vi "MGCC_FntStaMach_StateCalculandEnableFlagCalcul.vi"(7 "ABN State Input":string[](array[string]), 8 "Error Input":errorcluster[](array[cluster]), 9 "ABN State input enable":bool[][](array[boolean]), 10 "Current State":string[](array[string]), 11 "Input Events":bool[][](array[boolean])) -> (0 "Error output":errorcluster[](array[cluster]), 1 "Next State":string[](array[string]), 2 "ABN State output":string[](array[string]), 3 "ABN Function Enable output":bool[][](array[boolean]), 4 "Function Enable 2":bool[][](array[boolean]), 5 "Function Enable 1":bool[][](array[boolean]))   [LabVIEW 2016]
uses:
  MGCC_FntStaMach_gobal.vi
  <vilib>/imath/engines/lvmath2/RunTimeEngine/IndexRead/NIMS V(S).vi
  <instcachedir>/0/NIMS V(S)_0488751826AF41519A22953C041130DC.lvgen/NIMS V(S)_0488751826AF41519A22953C041130DC_003.vi
  <vilib>/imathl/engines/lvmath/Functions/Error Handling/Create Error.vi
  <vilib>/imath/engines/lvmath2/RunTimeEngine/NodeEndStatement/NIMS_NodeEndStatement_Output.vi
  <instcachedir>/0/NIMS_NodeEndStatement_Output_53EC0D466D134D7ABD903AC30B43404B.lvgen/NIMS_NodeEndStatement_Output_53EC0D466D134D7ABD903AC30B43404B_011.vi
  <vilib>/imath/engines/lvmath2/RunTimeEngine/ErrorHandling/NIMS_Finalize Error.vi
panel:
  out "error out":errorcluster
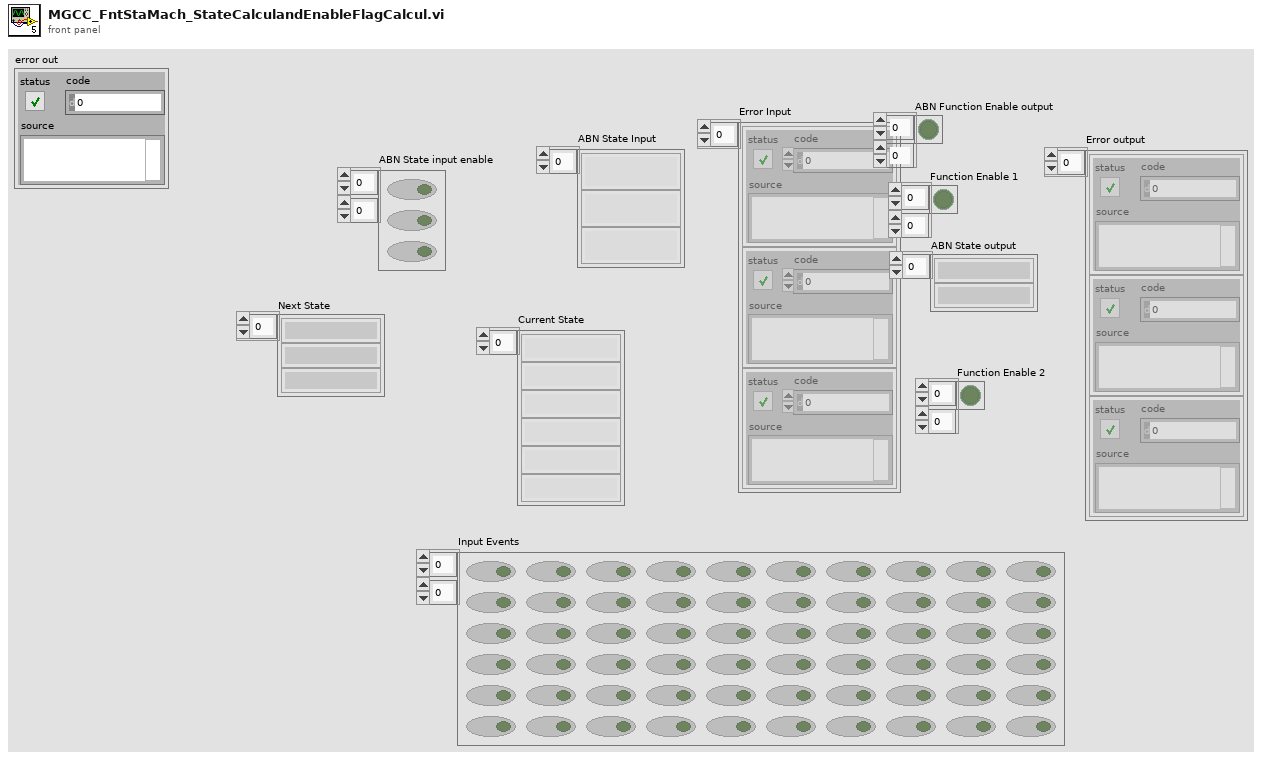
[diagram p1: front panel]
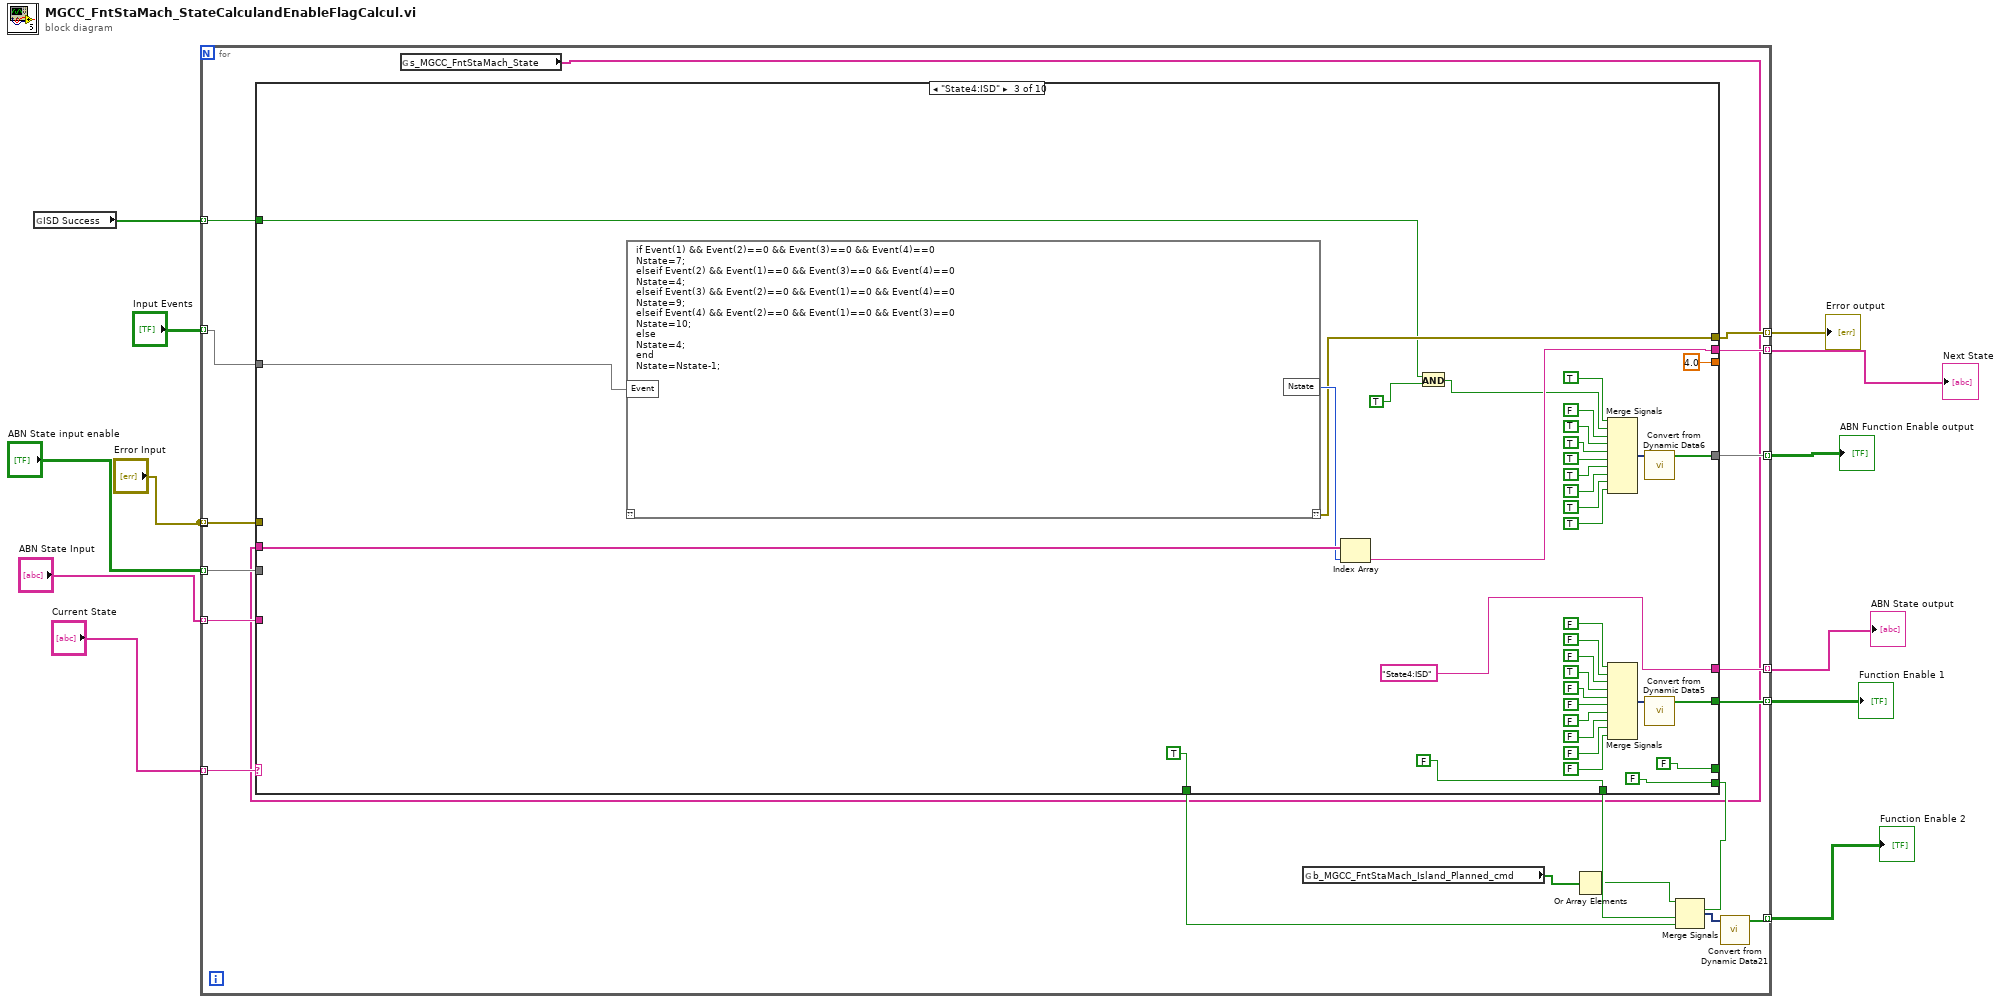
[diagram p0: block diagram]
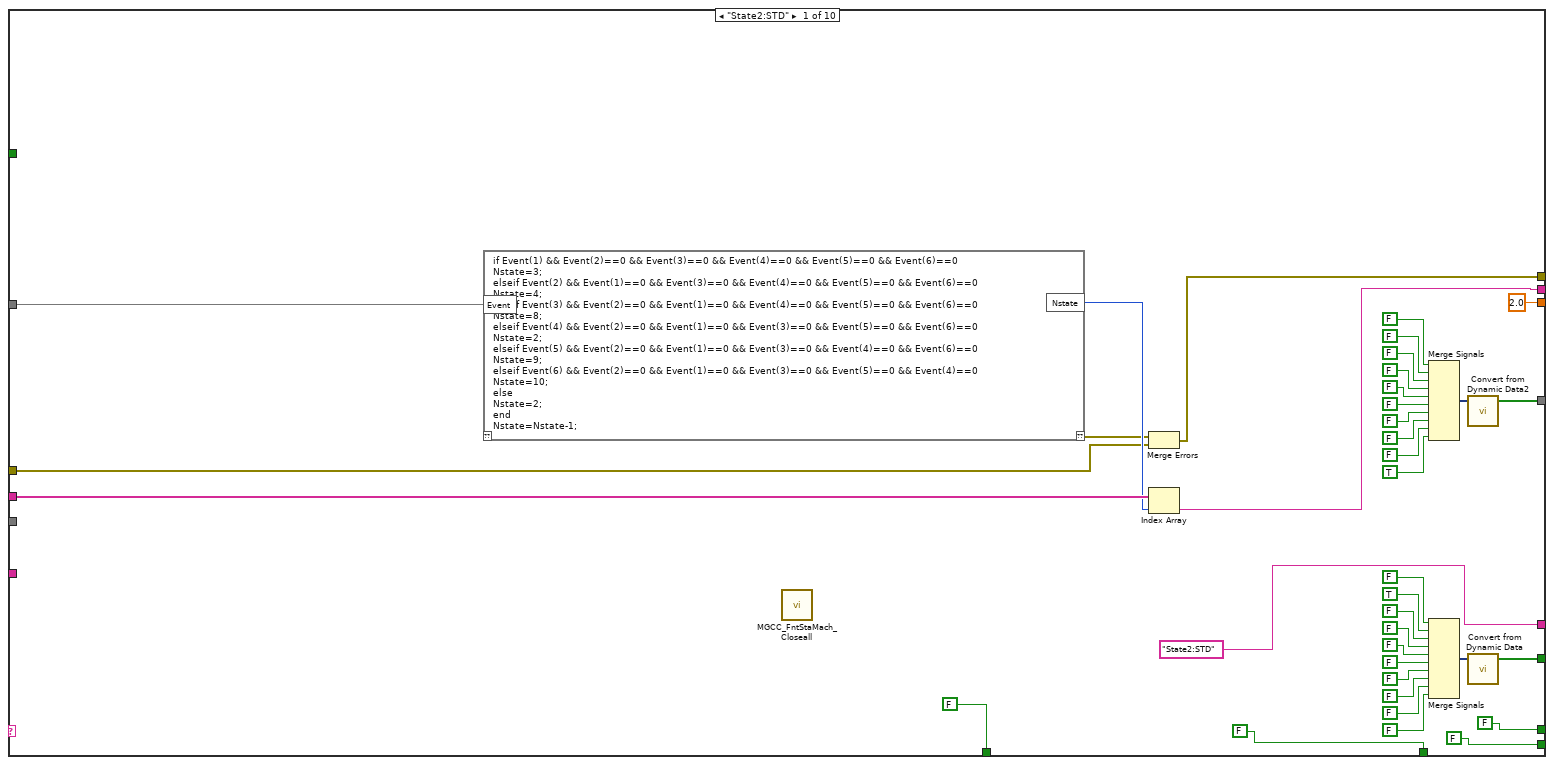
[diagram p2: hidden frame]
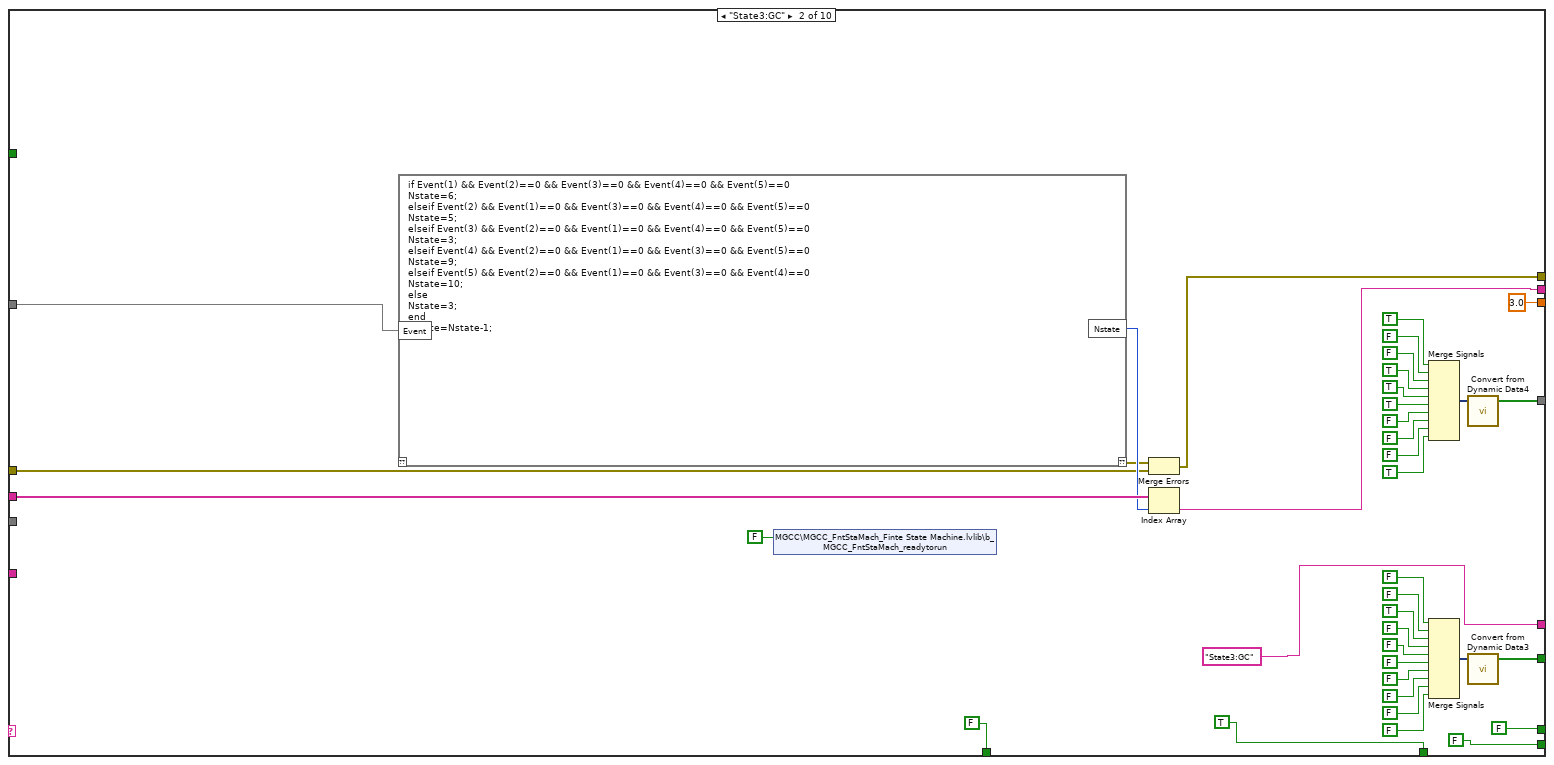
[diagram p3: hidden frame]
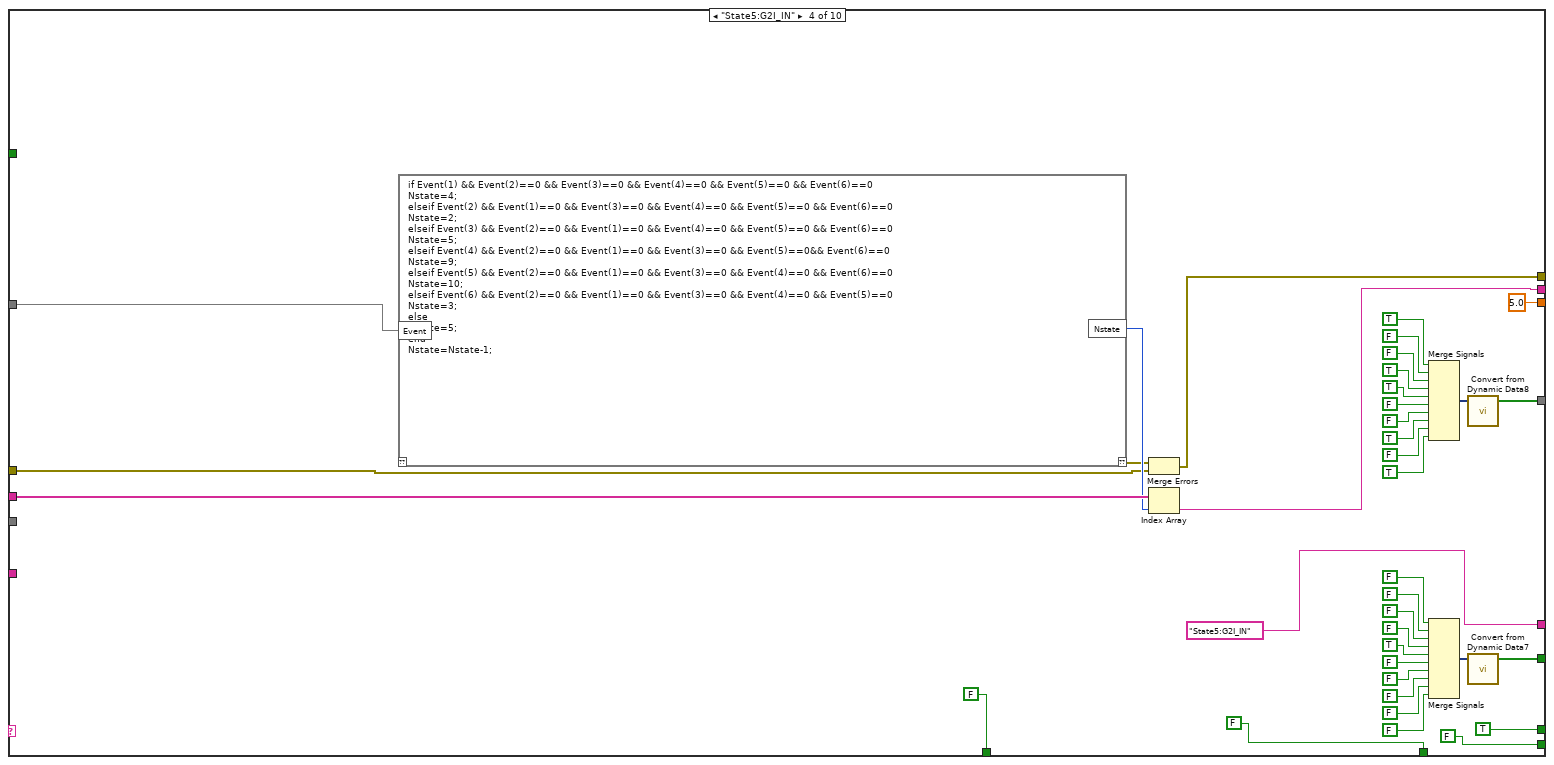
[diagram p4: hidden frame]
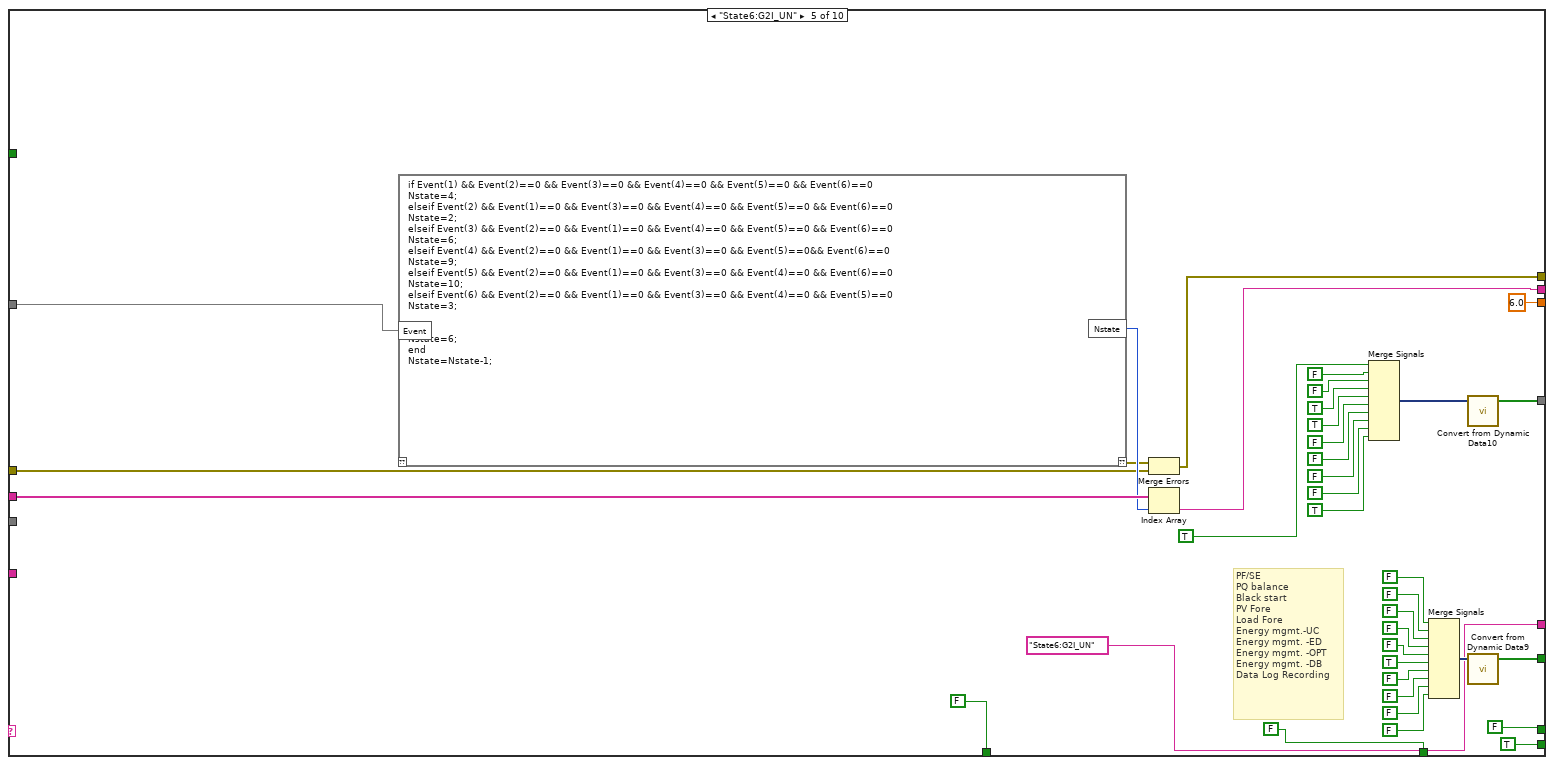
[diagram p5: hidden frame]
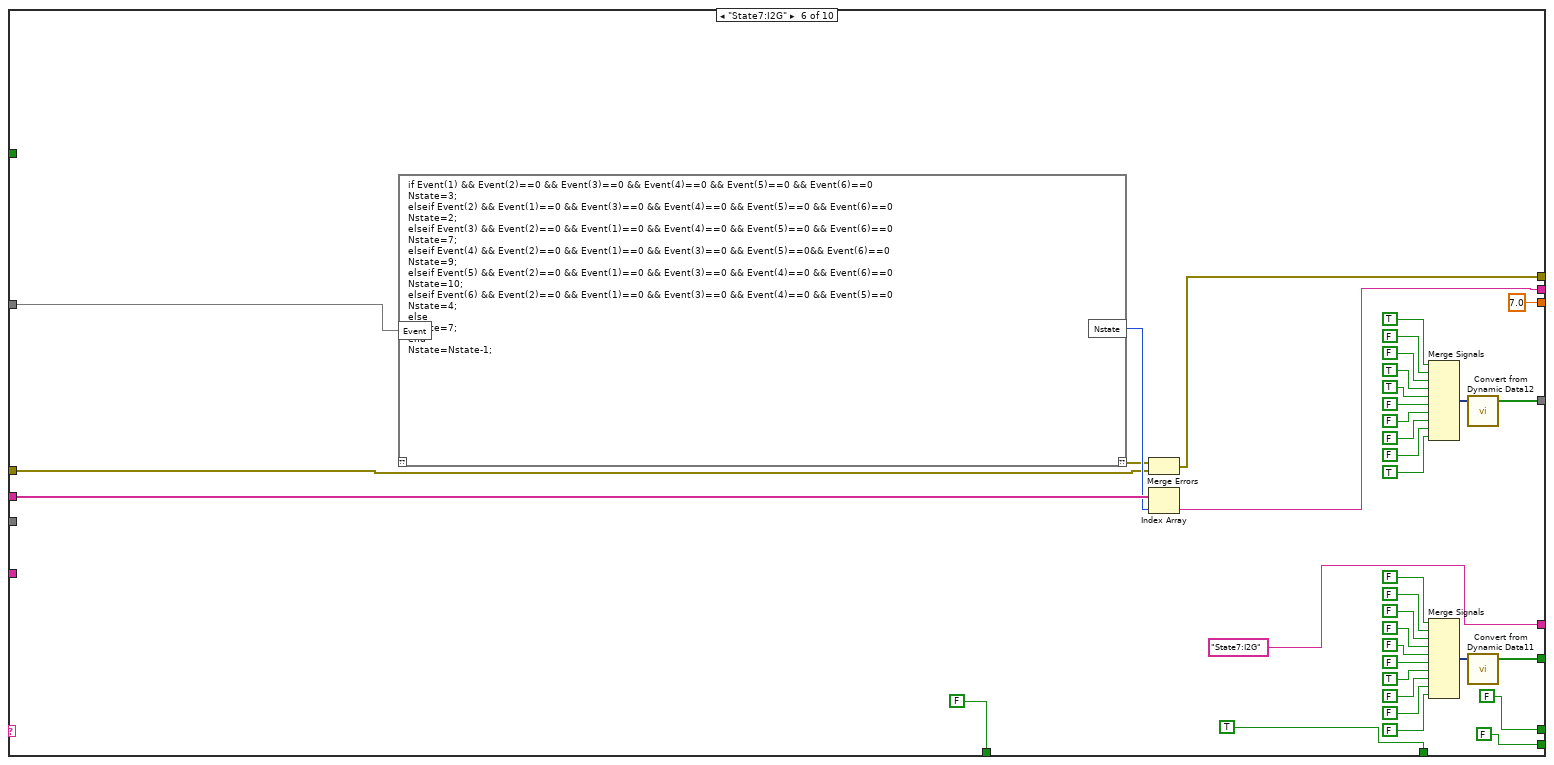
[diagram p6: hidden frame]
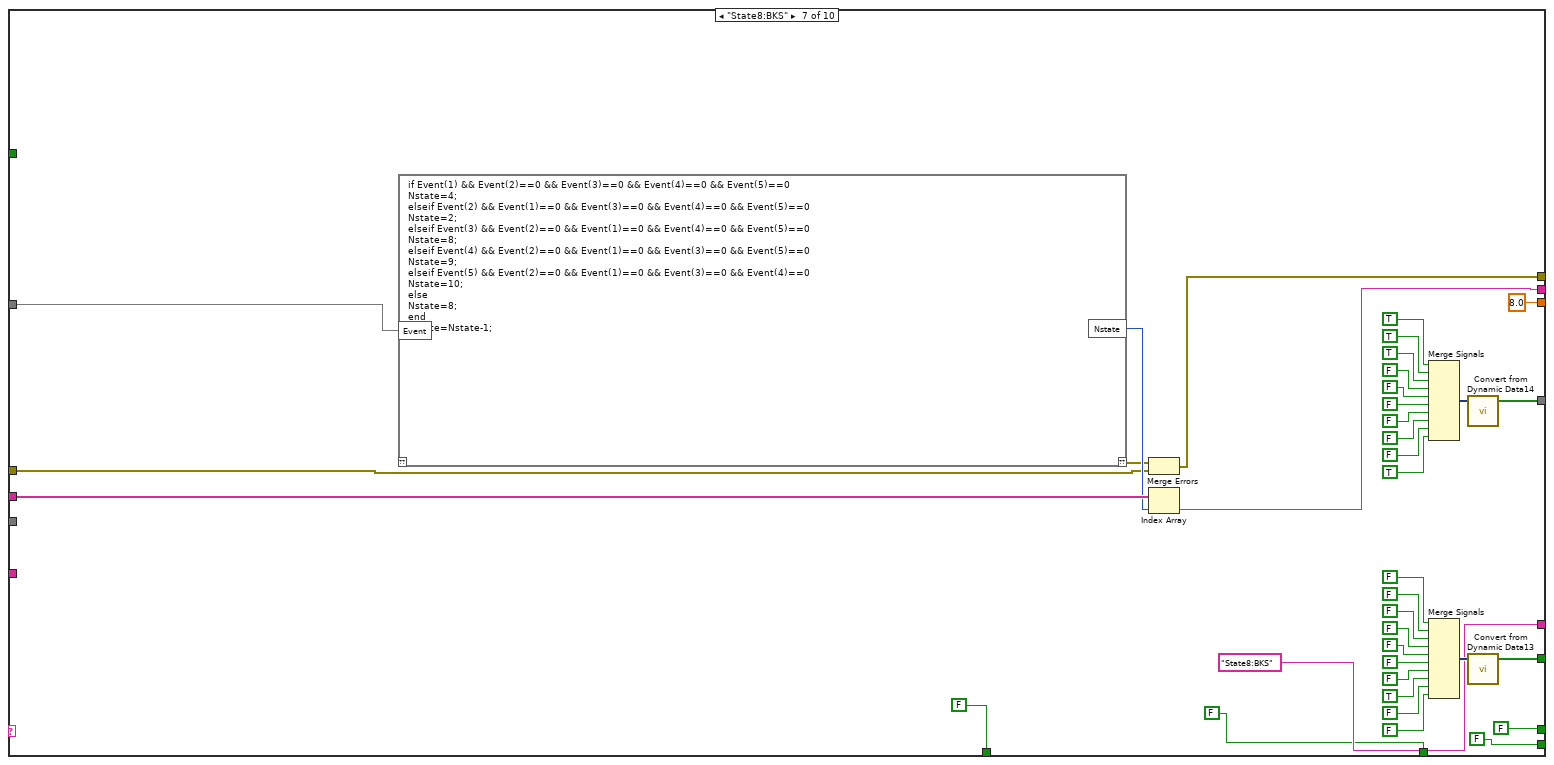
[diagram p7: hidden frame]
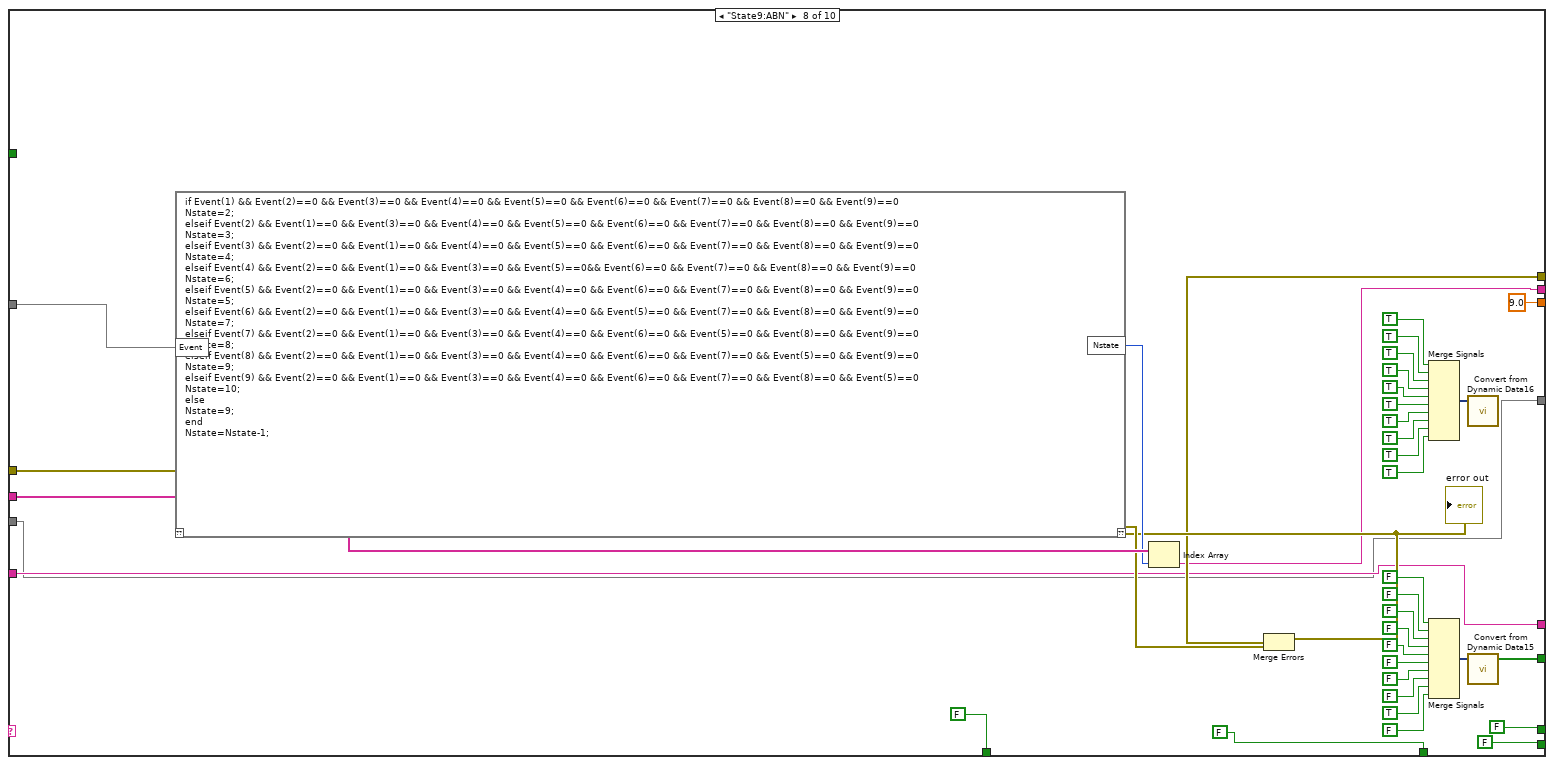
[diagram p8: hidden frame]
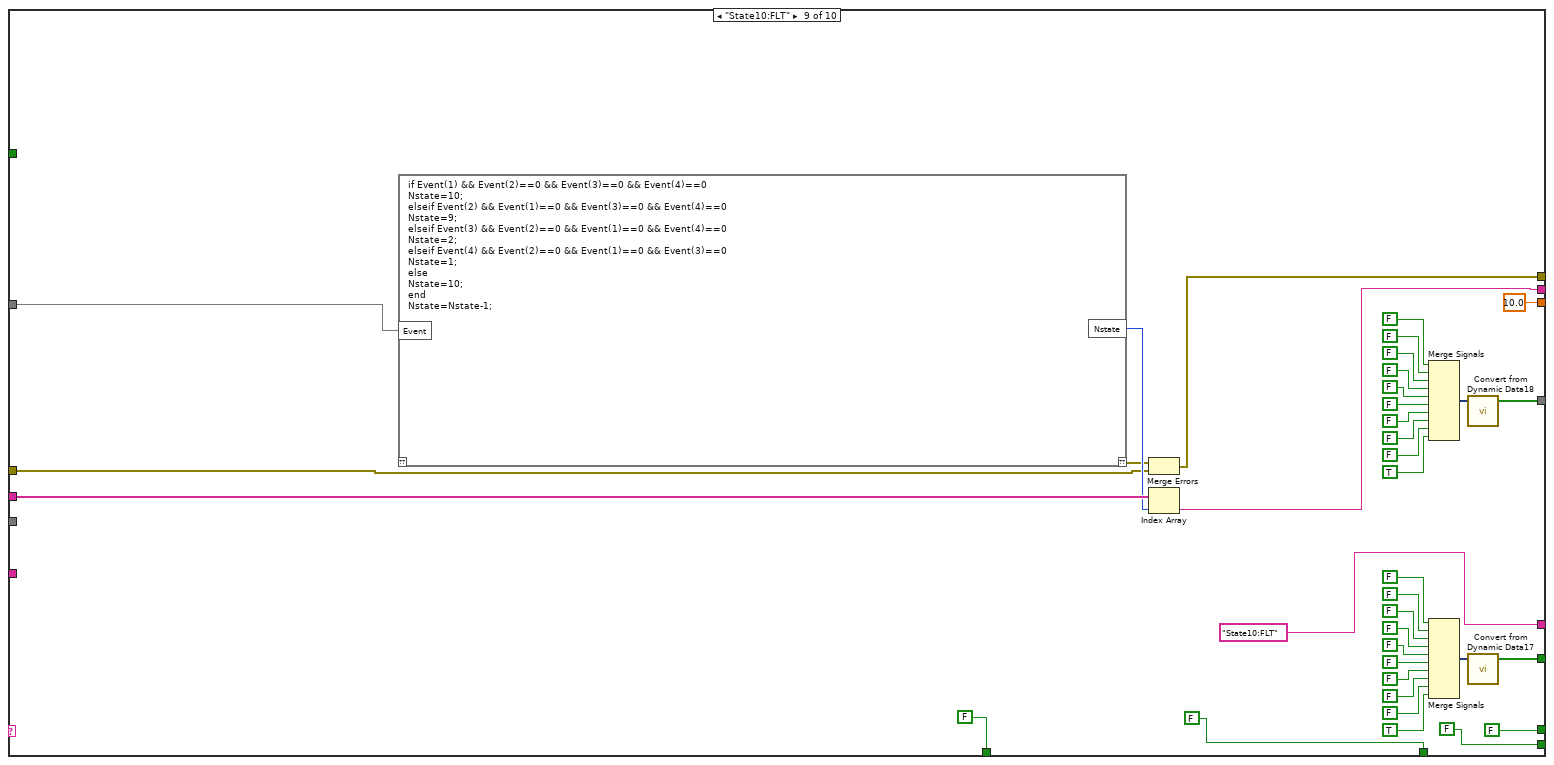
[diagram p9: hidden frame]
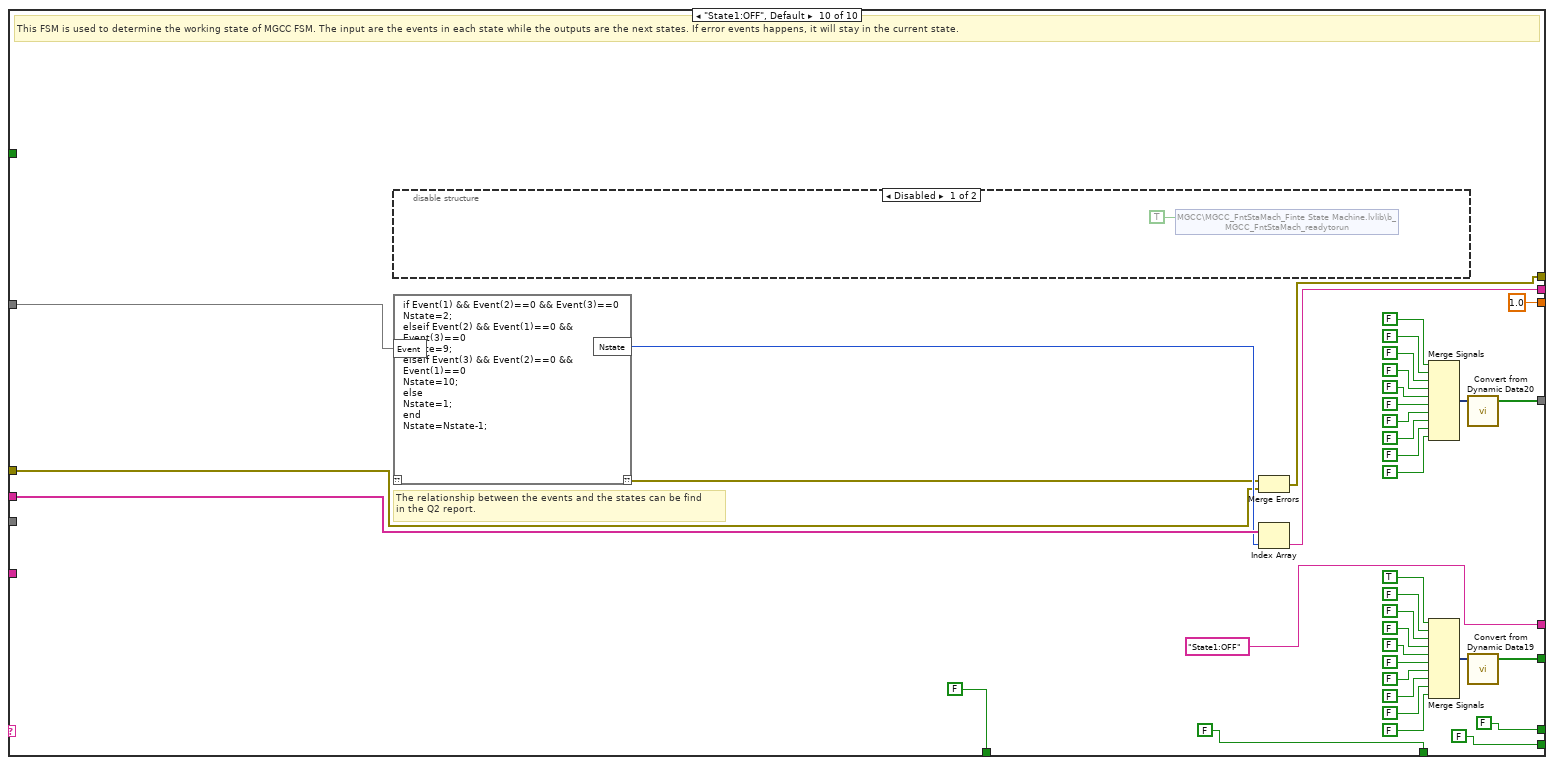
[diagram p10: hidden frame]
diagram:
  n1 = global read "MGCC_FntStaMach_gobal.vi" "ISD Success"() -> (w1:bool[])
  n2 = for {
    tunnel: "Input Events" -> [w30] mode=indexing
    tunnel: "Current State" -> [w31] mode=indexing
    tunnel: [w29] -> w10 mode=indexing
    tunnel: "Error Input" -> [_] mode=indexing
    tunnel: "Error Input" -> [w28] mode=indexing
    tunnel: [w27] -> w8 mode=indexing
    tunnel: [w26] -> w7 mode=indexing
    tunnel: "ABN State Input" -> [w25] mode=indexing
    tunnel: [w24] -> w5 mode=indexing
    tunnel: "ABN State input enable" -> [w23] mode=indexing
    tunnel: [w22] -> w3 mode=indexing
    tunnel: [w17] -> w2 mode=indexing
    tunnel: w1 -> [w15] mode=indexing
    n3 = global read "MGCC_FntStaMach_gobal.vi" "s_MGCC_FntStaMach_State"() -> (w16:string[])
    n4 = case shown="\"State4:ISD\"" w31 {
      tunnel: [w36 w1024 w1737 w2211 w3199 w4187 w5175 w5885 w8012 w8489] -> w22
      tunnel: [w57 w1046 w1754 w2232 w3220 w4208 w5196 w5904 w8032 w8510] -> w26
      tunnel: w16 -> [w56 w1045 w1753 w2231 w3219 w4207 w5195 w5903 w8031 w8509]
      tunnel: [w44 w1033 w1742 w2219 w3207 w4195 w5184 w5879 w8019 w8497] -> w27
      tunnel: [2.0 ("MS_Analog_Control_OS2_6") 3.0 ("MS_Analog_Control_OS2_6") 4.0 ("MS_Analog_Control_OS2_6") 5.0 ("MS_Analog_Control_OS2_6") 6.0 ("MS_Analog_Control_OS2_6") 7.0 ("MS_Analog_Control_OS2_6") 8.0 ("MS_Analog_Control_OS2_6") 9.0 ("MS_Analog_Control_OS2_6") 10.0 ("MS_Analog_Control_OS2_6") 1.0 ("MS_Analog_Control_OS2_6")] -> _
      tunnel: w30 -> [w41 w1029 w1739 w2216 w3204 w4192 w5180 w5889 w8016 w8494]
      tunnel: w28 -> [w40 w1028 _ w2215 w3203 w4191 w5179 w5888 w8015 w8493]
      tunnel: [w38 w1026 w1732 w2213 w3201 w4189 w5177 w5886 w8013 w8491] -> w29
      tunnel: ["State2:STD" "State3:GC" "State4:ISD" "State5:G2I_IN" "State6:G2I_UN" "State7:I2G" "State8:BKS" w5880 "State10:FLT" "State1:OFF"] -> w24
      tunnel: [FALSE ("State3") FALSE ("State3") FALSE ("State3") TRUE ("State3") FALSE ("State3") FALSE ("State3") FALSE ("State3") FALSE ("State3") FALSE ("State3") FALSE ("State3")] -> _
      tunnel: [FALSE ("State3") FALSE ("State3") FALSE ("State3") FALSE ("State3") TRUE ("State3") FALSE ("State3") FALSE ("State3") FALSE ("State3") FALSE ("State3") FALSE ("State3")] -> w21
      tunnel: [FALSE ("State3") TRUE ("State3") FALSE ("State3") FALSE ("State3") FALSE ("State3") TRUE ("State3") FALSE ("State3") FALSE ("State3") FALSE ("State3") FALSE ("State3")] -> w20
      tunnel: [FALSE ("State3") FALSE ("State3") TRUE ("State3") FALSE ("State3") FALSE ("State3") FALSE ("State3") FALSE ("State3") FALSE ("State3") FALSE ("State3") FALSE ("State3")] -> w19
      tunnel: w25 -> [_ _ _ _ _ _ _ w5880 _ _]
      tunnel: w23 -> [_ _ _ _ _ _ _ w5879 _ _]
      tunnel: w15 -> [_ _ w1731 _ _ _ _ _ _ _]
      frame "State2:STD" {
        n5 = mathscript code="if Event(1) && Event(2)==0 && Event(3)==0 && Event(4)==0 && Event(5)==0 && Event(6)==0\nNstate=3;\nelseif Event(2) && Event(1)==0 && Event(3)==0 && Event(4)==0 && Event(5)==0 && Event(6)==0\nNstate=4;\nelseif Event(3) && Event(2)==0 && Event(1)==0 && Event(4)==0 && Event(5)==0 && Event(6)==0\nNstate=8;\nelseif Event(4) && Event(2)==0 && Event(1)==0 && Event(3)==0 && Event(5)==0 && Event(6)==0\nNstate=2;\nelseif Event(5) && Event(2)==0 && Event(1)==0 && Event(3)==0 && Event(4)==0 && Event(6)==0\nNstate=9;\nelseif Event(6) && Event(2)==0 && Event(1)==0 && Event(3)==0 && Event(5)==0 && Event(4)==0\nNstate=10;\nelse\nNstate=2;\nend\nNstate=Nstate-1;"("Event"=w41) -> ("??"=w39:errorcluster, "Nstate"=w55:i32)  [unwired: 1 in]
        n6 = call "MGCC_FntStaMach_Closeall.vi"() -> ()  [unwired: 12 in]
        n7 = Merge Errors(w39, w40) -> (w38:errorcluster)
        n8 = Index Array(array=w56, index=w55) -> (element=w36:string)
        n9 = Merge Signals(FALSE ("State3"), FALSE ("State3"), FALSE ("State3"), FALSE ("State3"), FALSE ("State3"), FALSE ("State3"), FALSE ("State3"), FALSE ("State3"), FALSE ("State3"), TRUE ("State3")) -> (w45:dynamicdata)
        n10 = Merge Signals(FALSE ("State3"), TRUE ("State3"), FALSE ("State3"), FALSE ("State3"), FALSE ("State3"), FALSE ("State3"), FALSE ("State3"), FALSE ("State3"), FALSE ("State3"), FALSE ("State3")) -> (w58:dynamicdata)
        n11 = call "Convert from Dynamic Data2"("Dynamic Data Type"=w45) -> ("Array"=w44:bool[])  [unwired: 3 in]
        n12 = call "Convert from Dynamic Data"("Dynamic Data Type"=w58) -> ("Array"=w57:bool[])  [unwired: 3 in]
      }
      frame "State3:GC" {
        n13 = mathscript code="if Event(1) && Event(2)==0 && Event(3)==0 && Event(4)==0 && Event(5)==0 \nNstate=6;\nelseif Event(2) && Event(1)==0 && Event(3)==0 && Event(4)==0 && Event(5)==0 \nNstate=5;\nelseif Event(3) && Event(2)==0 && Event(1)==0 && Event(4)==0 && Event(5)==0 \nNstate=3;\nelseif Event(4) && Event(2)==0 && Event(1)==0 && Event(3)==0 && Event(5)==0\nNstate=9;\nelseif Event(5) && Event(2)==0 && Event(1)==0 && Event(3)==0 && Event(4)==0 \nNstate=10;\nelse\nNstate=3;\nend\nNstate=Nstate-1;"("Event"=w1029) -> ("??"=w1027:errorcluster, "Nstate"=w1044:i32)  [unwired: 1 in]
        n14 = shared-variable "MGCC\\MGCC_FntStaMach_Finte State Machine.lvlib\\b_MGCC_FntStaMach_readytorun"(FALSE ("b_MGCC_DataLog_enable")) -> ()  [unwired: 1 in, 1 out]
        n15 = Merge Errors(w1027, w1028) -> (w1026:errorcluster)
        n16 = Index Array(array=w1045, index=w1044) -> (element=w1024:string)
        n17 = Merge Signals(TRUE ("State3"), FALSE ("State3"), FALSE ("State3"), TRUE ("State3"), TRUE ("State3"), TRUE ("State3"), FALSE ("State3"), FALSE ("State3"), FALSE ("State3"), TRUE ("State3")) -> (w1034:dynamicdata)
        n18 = Merge Signals(FALSE ("State3"), FALSE ("State3"), TRUE ("State3"), FALSE ("State3"), FALSE ("State3"), FALSE ("State3"), FALSE ("State3"), FALSE ("State3"), FALSE ("State3"), FALSE ("State3")) -> (w1047:dynamicdata)
        n19 = call "Convert from Dynamic Data4"("Dynamic Data Type"=w1034) -> ("Array"=w1033:bool[])  [unwired: 3 in]
        n20 = call "Convert from Dynamic Data3"("Dynamic Data Type"=w1047) -> ("Array"=w1046:bool[])  [unwired: 3 in]
      }
      frame "State4:ISD" {
        n21 = mathscript code="if Event(1) && Event(2)==0 && Event(3)==0 && Event(4)==0 \nNstate=7;\nelseif Event(2) && Event(1)==0 && Event(3)==0 && Event(4)==0 \nNstate=4;\nelseif Event(3) && Event(2)==0 && Event(1)==0 && Event(4)==0 \nNstate=9;\nelseif Event(4) && Event(2)==0 && Event(1)==0 && Event(3)==0 \nNstate=10;\nelse\nNstate=4;\nend\nNstate=Nstate-1;"("Event"=w1739) -> ("??"=w1732:errorcluster, "Nstate"=w1752:i32)  [unwired: 1 in]
        n22 = Index Array(array=w1753, index=w1752) -> (element=w1737:string)
        n23 = And(x=w1731, y=TRUE ("State3")) -> (x .and. y?=w1729:bool)
        n24 = Merge Signals(TRUE ("State3"), w1729, FALSE ("State3"), TRUE ("State3"), TRUE ("State3"), TRUE ("State3"), TRUE ("State3"), TRUE ("State3"), TRUE ("State3"), TRUE ("State3")) -> (w1743:dynamicdata)
        n25 = Merge Signals(FALSE ("State3"), FALSE ("State3"), FALSE ("State3"), TRUE ("State3"), FALSE ("State3"), FALSE ("State3"), FALSE ("State3"), FALSE ("State3"), FALSE ("State3"), FALSE ("State3")) -> (w1755:dynamicdata)
        n26 = call "Convert from Dynamic Data6"("Dynamic Data Type"=w1743) -> ("Array"=w1742:bool[])  [unwired: 3 in]
        n27 = call "Convert from Dynamic Data5"("Dynamic Data Type"=w1755) -> ("Array"=w1754:bool[])  [unwired: 3 in]
      }
      frame "State5:G2I_IN" {
        n28 = mathscript code="if Event(1) && Event(2)==0 && Event(3)==0 && Event(4)==0 && Event(5)==0 && Event(6)==0\nNstate=4;\nelseif Event(2) && Event(1)==0 && Event(3)==0 && Event(4)==0 && Event(5)==0 && Event(6)==0\nNstate=2;\nelseif Event(3) && Event(2)==0 && Event(1)==0 && Event(4)==0 && Event(5)==0 && Event(6)==0\nNstate=5;\nelseif Event(4) && Event(2)==0 && Event(1)==0 && Event(3)==0 && Event(5)==0&& Event(6)==0\nNstate=9;\nelseif Event(5) && Event(2)==0 && Event(1)==0 && Event(3)==0 && Event(4)==0 && Event(6)==0\nNstate=10;\nelseif Event(6) && Event(2)==0 && Event(1)==0 && Event(3)==0 && Event(4)==0 && Event(5)==0\nNstate=3;\nelse\nNstate=5;\nend\nNstate=Nstate-1;"("Event"=w2216) -> ("??"=w2214:errorcluster, "Nstate"=w2230:i32)  [unwired: 1 in]
        n29 = Merge Errors(w2214, w2215) -> (w2213:errorcluster)
        n30 = Index Array(array=w2231, index=w2230) -> (element=w2211:string)
        n31 = Merge Signals(TRUE ("State3"), FALSE ("State3"), FALSE ("State3"), TRUE ("State3"), TRUE ("State3"), FALSE ("State3"), FALSE ("State3"), TRUE ("State3"), FALSE ("State3"), TRUE ("State3")) -> (w2220:dynamicdata)
        n32 = Merge Signals(FALSE ("State3"), FALSE ("State3"), FALSE ("State3"), FALSE ("State3"), TRUE ("State3"), FALSE ("State3"), FALSE ("State3"), FALSE ("State3"), FALSE ("State3"), FALSE ("State3")) -> (w2233:dynamicdata)
        n33 = call "Convert from Dynamic Data8"("Dynamic Data Type"=w2220) -> ("Array"=w2219:bool[])  [unwired: 3 in]
        n34 = call "Convert from Dynamic Data7"("Dynamic Data Type"=w2233) -> ("Array"=w2232:bool[])  [unwired: 3 in]
      }
      frame "State6:G2I_UN" {
        # "PF/SE\nPQ balance\nBlack start\nPV Fore\nLoad Fore\nEnergy mgmt.-UC\nEnergy mgmt. -ED\nEnergy mgmt. -OPT\nEnergy mgmt. -DB\nData Log Recording"
        n35 = mathscript code="if Event(1) && Event(2)==0 && Event(3)==0 && Event(4)==0 && Event(5)==0 && Event(6)==0\nNstate=4;\nelseif Event(2) && Event(1)==0 && Event(3)==0 && Event(4)==0 && Event(5)==0 && Event(6)==0\nNstate=2;\nelseif Event(3) && Event(2)==0 && Event(1)==0 && Event(4)==0 && Event(5)==0 && Event(6)==0\nNstate=6;\nelseif Event(4) && Event(2)==0 && Event(1)==0 && Event(3)==0 && Event(5)==0&& Event(6)==0\nNstate=9;\nelseif Event(5) && Event(2)==0 && Event(1)==0 && Event(3)==0 && Event(4)==0 && Event(6)==0\nNstate=10;\nelseif Event(6) && Event(2)==0 && Event(1)==0 && Event(3)==0 && Event(4)==0 && Event(5)==0\nNstate=3;\n\nelse\nNstate=6;\nend\nNstate=Nstate-1;"("Event"=w3204) -> ("??"=w3202:errorcluster, "Nstate"=w3218:i32)  [unwired: 1 in]
        n36 = Merge Errors(w3202, w3203) -> (w3201:errorcluster)
        n37 = Index Array(array=w3219, index=w3218) -> (element=w3199:string)
        n38 = Merge Signals(TRUE ("State3"), FALSE ("State3"), FALSE ("State3"), TRUE ("State3"), TRUE ("State3"), FALSE ("State3"), FALSE ("State3"), FALSE ("State3"), FALSE ("State3"), TRUE ("State3")) -> (w3208:dynamicdata)
        n39 = Merge Signals(FALSE ("State3"), FALSE ("State3"), FALSE ("State3"), FALSE ("State3"), FALSE ("State3"), TRUE ("State3"), FALSE ("State3"), FALSE ("State3"), FALSE ("State3"), FALSE ("State3")) -> (w3221:dynamicdata)
        n40 = call "Convert from Dynamic Data10"("Dynamic Data Type"=w3208) -> ("Array"=w3207:bool[])  [unwired: 3 in]
        n41 = call "Convert from Dynamic Data9"("Dynamic Data Type"=w3221) -> ("Array"=w3220:bool[])  [unwired: 3 in]
      }
      frame "State7:I2G" {
        n42 = mathscript code="if Event(1) && Event(2)==0 && Event(3)==0 && Event(4)==0 && Event(5)==0 && Event(6)==0 \nNstate=3;\nelseif Event(2) && Event(1)==0 && Event(3)==0 && Event(4)==0 && Event(5)==0 && Event(6)==0 \nNstate=2;\nelseif Event(3) && Event(2)==0 && Event(1)==0 && Event(4)==0 && Event(5)==0 && Event(6)==0 \nNstate=7;\nelseif Event(4) && Event(2)==0 && Event(1)==0 && Event(3)==0 && Event(5)==0&& Event(6)==0 \nNstate=9;\nelseif Event(5) && Event(2)==0 && Event(1)==0 && Event(3)==0 && Event(4)==0 && Event(6)==0 \nNstate=10;\nelseif Event(6) && Event(2)==0 && Event(1)==0 && Event(3)==0 && Event(4)==0 && Event(5)==0 \nNstate=4;\nelse\nNstate=7;\nend\nNstate=Nstate-1;"("Event"=w4192) -> ("??"=w4190:errorcluster, "Nstate"=w4206:i32)  [unwired: 1 in]
        n43 = Merge Errors(w4190, w4191) -> (w4189:errorcluster)
        n44 = Index Array(array=w4207, index=w4206) -> (element=w4187:string)
        n45 = Merge Signals(TRUE ("State3"), FALSE ("State3"), FALSE ("State3"), TRUE ("State3"), TRUE ("State3"), FALSE ("State3"), FALSE ("State3"), FALSE ("State3"), FALSE ("State3"), TRUE ("State3")) -> (w4196:dynamicdata)
        n46 = Merge Signals(FALSE ("State3"), FALSE ("State3"), FALSE ("State3"), FALSE ("State3"), FALSE ("State3"), FALSE ("State3"), TRUE ("State3"), FALSE ("State3"), FALSE ("State3"), FALSE ("State3")) -> (w4209:dynamicdata)
        n47 = call "Convert from Dynamic Data12"("Dynamic Data Type"=w4196) -> ("Array"=w4195:bool[])  [unwired: 3 in]
        n48 = call "Convert from Dynamic Data11"("Dynamic Data Type"=w4209) -> ("Array"=w4208:bool[])  [unwired: 3 in]
      }
      frame "State8:BKS" {
        n49 = mathscript code="if Event(1) && Event(2)==0 && Event(3)==0 && Event(4)==0 && Event(5)==0 \nNstate=4;\nelseif Event(2) && Event(1)==0 && Event(3)==0 && Event(4)==0 && Event(5)==0 \nNstate=2;\nelseif Event(3) && Event(2)==0 && Event(1)==0 && Event(4)==0 && Event(5)==0 \nNstate=8;\nelseif Event(4) && Event(2)==0 && Event(1)==0 && Event(3)==0 && Event(5)==0\nNstate=9;\nelseif Event(5) && Event(2)==0 && Event(1)==0 && Event(3)==0 && Event(4)==0 \nNstate=10;\nelse\nNstate=8;\nend\nNstate=Nstate-1;"("Event"=w5180) -> ("??"=w5178:errorcluster, "Nstate"=w5181:i32)  [unwired: 1 in]
        n50 = Merge Errors(w5178, w5179) -> (w5177:errorcluster)
        n51 = Index Array(array=w5195, index=w5181) -> (element=w5175:string)
        n52 = Merge Signals(TRUE ("State3"), TRUE ("State3"), TRUE ("State3"), FALSE ("State3"), FALSE ("State3"), FALSE ("State3"), FALSE ("State3"), FALSE ("State3"), FALSE ("State3"), TRUE ("State3")) -> (w5185:dynamicdata)
        n53 = Merge Signals(FALSE ("State3"), FALSE ("State3"), FALSE ("State3"), FALSE ("State3"), FALSE ("State3"), FALSE ("State3"), FALSE ("State3"), TRUE ("State3"), FALSE ("State3"), FALSE ("State3")) -> (w5197:dynamicdata)
        n54 = call "Convert from Dynamic Data14"("Dynamic Data Type"=w5185) -> ("Array"=w5184:bool[])  [unwired: 3 in]
        n55 = call "Convert from Dynamic Data13"("Dynamic Data Type"=w5197) -> ("Array"=w5196:bool[])  [unwired: 3 in]
      }
      frame "State9:ABN" {
        n56 = mathscript code="if Event(1) && Event(2)==0 && Event(3)==0 && Event(4)==0 && Event(5)==0 && Event(6)==0 && Event(7)==0 && Event(8)==0 && Event(9)==0 \nNstate=2;\nelseif Event(2) && Event(1)==0 && Event(3)==0 && Event(4)==0 && Event(5)==0 && Event(6)==0 && Event(7)==0 && Event(8)==0 && Event(9)==0 \nNstate=3;\nelseif Event(3) && Event(2)==0 && Event(1)==0 && Event(4)==0 && Event(5)==0 && Event(6)==0 && Event(7)==0 && Event(8)==0 && Event(9)==0 \nNstate=4;\nelseif Event(4) && Event(2)==0 && Event(1)==0 && Event(3)==0 && Event(5)==0&& Event(6)==0 && Event(7)==0 && Event(8)==0 && Event(9)==0 \nNstate=6;\nelseif Event(5) && Event(2)==0 && Event(1)==0 && Event(3)==0 && Event(4)==0 && Event(6)==0 && Event(7)==0 && Event(8)==0 && Event(9)==0 \nNstate=5;\nelseif Event(6) && Event(2)==0 && Event(1)==0 && Event(3)==0 && Event(4)==0 && Event(5)==0 && Event(7)==0 && Event(8)==0 && Event(9)==0 \nNstate=7;\nelseif Event(7) && Event(2)==0 && Event(1)==0 && Event(3)==0 && Event(4)==0 && Event(6)==0 && Event(5)==0 && Event(8)==0 && Event(9)==0 \nNstate=8;\nelseif Event(8) && Event(2)==0 && Event(1)==0 && Event(3)==0 && Event(4)==0 && Event(6)==0 && Event(7)==0 && Event(5)==0 && Event(9)==0 \nNstate=9;\nelseif Event(9) && Event(2)==0 && Event(1)==0 && Event(3)==0 && Event(4)==0 && Event(6)==0 && Event(7)==0 && Event(8)==0 && Event(5)==0 \nNstate=10;\nelse\nNstate=9;\nend\nNstate=Nstate-1;"("Event"=w5889) -> ("??"=w5887:errorcluster, "Nstate"=w5902:i32)  [unwired: 1 in]
        "error out" <- w5887
        n57 = Index Array(array=w5903, index=w5902) -> (element=w5885:string)
        n58 = Merge Errors(w5887, w5888) -> (w5886:errorcluster)
        n59 = Merge Signals(TRUE ("State3"), TRUE ("State3"), TRUE ("State3"), TRUE ("State3"), TRUE ("State3"), TRUE ("State3"), TRUE ("State3"), TRUE ("State3"), TRUE ("State3"), TRUE ("State3")) -> (w5892:dynamicdata)
        n60 = Merge Signals(FALSE ("State3"), FALSE ("State3"), FALSE ("State3"), FALSE ("State3"), FALSE ("State3"), FALSE ("State3"), FALSE ("State3"), FALSE ("State3"), TRUE ("State3"), FALSE ("State3")) -> (w5905:dynamicdata)
        n61 = call "Convert from Dynamic Data16"("Dynamic Data Type"=w5892) -> ()  [unwired: 3 in, 1 out]
        n62 = call "Convert from Dynamic Data15"("Dynamic Data Type"=w5905) -> ("Array"=w5904:bool[])  [unwired: 3 in]
      }
      frame "State10:FLT" {
        n63 = mathscript code="if Event(1) && Event(2)==0 && Event(3)==0 && Event(4)==0 \nNstate=10;\nelseif Event(2) && Event(1)==0 && Event(3)==0 && Event(4)==0 \nNstate=9;\nelseif Event(3) && Event(2)==0 && Event(1)==0 && Event(4)==0 \nNstate=2;\nelseif Event(4) && Event(2)==0 && Event(1)==0 && Event(3)==0 \nNstate=1;\nelse\nNstate=10;\nend\nNstate=Nstate-1;"("Event"=w8016) -> ("??"=w8014:errorcluster, "Nstate"=w8030:i32)  [unwired: 1 in]
        n64 = Merge Errors(w8014, w8015) -> (w8013:errorcluster)
        n65 = Index Array(array=w8031, index=w8030) -> (element=w8012:string)
        n66 = Merge Signals(FALSE ("State3"), FALSE ("State3"), FALSE ("State3"), FALSE ("State3"), FALSE ("State3"), FALSE ("State3"), FALSE ("State3"), FALSE ("State3"), FALSE ("State3"), TRUE ("State3")) -> (w8020:dynamicdata)
        n67 = Merge Signals(FALSE ("State3"), FALSE ("State3"), FALSE ("State3"), FALSE ("State3"), FALSE ("State3"), FALSE ("State3"), FALSE ("State3"), FALSE ("State3"), FALSE ("State3"), TRUE ("State3")) -> (w8033:dynamicdata)
        n68 = call "Convert from Dynamic Data18"("Dynamic Data Type"=w8020) -> ("Array"=w8019:bool[])  [unwired: 3 in]
        n69 = call "Convert from Dynamic Data17"("Dynamic Data Type"=w8033) -> ("Array"=w8032:bool[])  [unwired: 3 in]
      }
      frame "State1:OFF", Default {
        # "The relationship between the events and the states can be find\nin the Q2 report."
        # "This FSM is used to determine the working state of MGCC FSM. The input are the events in each state while the outputs are the next states. If error events happens, it will stay in the current state."
        n70 = disable-structure shown="Disabled" {
          frame Disabled {
            n71 = shared-variable "MGCC\\MGCC_FntStaMach_Finte State Machine.lvlib\\b_MGCC_FntStaMach_readytorun"(TRUE ("b_MGCC_DataLog_enable")) -> ()  [unwired: 1 in, 1 out]
          }
          frame Enabled {
          }
        }
        n72 = mathscript code="if Event(1) && Event(2)==0 && Event(3)==0\nNstate=2;\nelseif Event(2) && Event(1)==0 && Event(3)==0\nNstate=9;\nelseif Event(3) && Event(2)==0 && Event(1)==0\nNstate=10;\nelse\nNstate=1;\nend\nNstate=Nstate-1;"("Event"=w8494) -> ("??"=w8492:errorcluster, "Nstate"=w8508:i32)  [unwired: 1 in]
        n73 = Merge Errors(w8492, w8493) -> (w8491:errorcluster)
        n74 = Index Array(array=w8509, index=w8508) -> (element=w8489:string)
        n75 = Merge Signals(FALSE ("State3"), FALSE ("State3"), FALSE ("State3"), FALSE ("State3"), FALSE ("State3"), FALSE ("State3"), FALSE ("State3"), FALSE ("State3"), FALSE ("State3"), FALSE ("State3")) -> (w8498:dynamicdata)
        n76 = Merge Signals(TRUE ("State3"), FALSE ("State3"), FALSE ("State3"), FALSE ("State3"), FALSE ("State3"), FALSE ("State3"), FALSE ("State3"), FALSE ("State3"), FALSE ("State3"), FALSE ("State3")) -> (w8511:dynamicdata)
        n77 = call "Convert from Dynamic Data20"("Dynamic Data Type"=w8498) -> ("Array"=w8497:bool[])  [unwired: 3 in]
        n78 = call "Convert from Dynamic Data19"("Dynamic Data Type"=w8511) -> ("Array"=w8510:bool[])  [unwired: 3 in]
      }
    }
    n79 = global read "MGCC_FntStaMach_gobal.vi" "b_MGCC_FntStaMach_Island_Planned_cmd"() -> (w14:bool[])
    n80 = Or Array Elements(Boolean array=w14) -> (logical OR=w13:bool)
    n81 = Merge Signals(w13, w21, w20, w19) -> (w18:dynamicdata)
    n82 = call "Convert from Dynamic Data21"("Dynamic Data Type"=w18) -> ("Array"=w17:bool[])  [unwired: 3 in]
  }
  "Error output" <- w10
  "ABN Function Enable output" <- w8
  "Function Enable 1" <- w7
  "ABN State output" <- w5
  "Next State" <- w3
  "Function Enable 2" <- w2
